vi "Create Object.vi"(8 "error in (no error)":errorcluster, 10 "Object Name":string, 11 "CS++Factory in":refnum<class "CS++Factory.lvclass">) -> (0 "error out":errorcluster, 1 "Attributes found?":bool, 2 "LabVIEW Object":refnum<class>, 3 "CS++Factory out":refnum<class "CS++Factory.lvclass">)   [LabVIEW 2013, in "CS++BaseClasses.lvlib" / "CS++Factory.lvclass"]
doc: "Create an object by name. Object name is a kind of reference to attribute initialization data."
uses:
  CS++Factory.lvclass
  Base/CS++Base.lvclass
  Actors/CS++BaseActor/CS++BaseActor.lvclass
  Actors/CS++BaseActor/CS++BaseActor.lvclass/CS++BaseActor.ctl
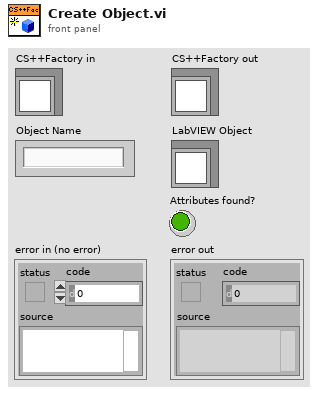
[diagram p1: front panel]
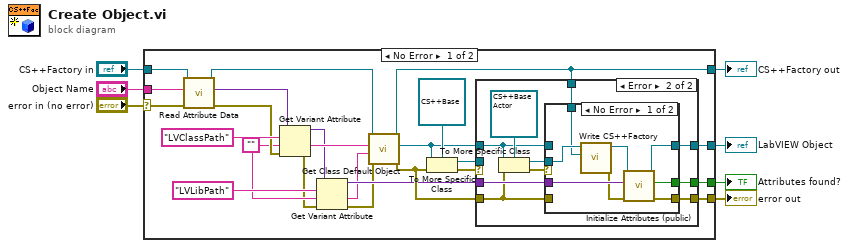
[diagram p0: block diagram]
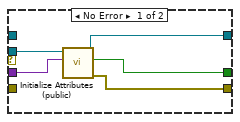
[diagram p2: hidden frame]
diagram:
  n1 = case shown="No Error" "error in (no error)" {
    selector: "error in (no error)" -> [w22 w58]
    tunnel: [w23 w58] -> w6
    tunnel: [w18 w57] -> w4
    tunnel: "CS++Factory in" -> [w31 w57]
    tunnel: [w24 _] -> w3
    tunnel: "Object Name" -> [w30 _]
    tunnel: [w21 _] -> w1
    frame No Error {
      w10 = ""
      n2 = call-dynamic "Read Attribute Data.vi"("error in (no error)"=w22, "Object Name"=w30, "CS++Factory in"=w31) -> ("error out"=w27:errorcluster, "Attribute Data"=w29:variant, "CS++Factory out"=w19:refnum<class "CS++Factory.lvclass">)  [unwired: 6 in]
      n3 = Get Variant Attribute(Variant=w29, name="LVClassPath", default value (empty Variant)=w10, error in=w27) -> (duplicate Variant=w13:variant, value=w16:string, error out=w9:errorcluster)  [unwired: 1 out]
      n4 = Get Variant Attribute(Variant=w13, name="LVLibPath", default value (empty Variant)=w10, error in=w9) -> (duplicate Variant=w12:variant, value=w11:string, error out=w8:errorcluster)  [unwired: 1 out]
      n5 = call-dynamic "Get Class Default Object.vi"("error in (no error)"=w8, "Library Path/Name"=w11, "Class Path/Name"=w16, "CS++Factory in"=w19) -> ("error out"=w17:errorcluster, "Class Default Object"=w15:refnum<class>, "CS++Factory out"=w18:refnum<class "CS++Factory.lvclass">)  [unwired: 5 in]
      n6 = To More Specific Class(target class=refnum<class "CS++Base.lvclass"> refnum ("CS++BaseClasses.lvlib:CS++Base.lvclass"), reference=w15, error in=w17) -> (specific class reference=w25:refnum<class "CS++Base.lvclass">, error out=w20:errorcluster)
      n7 = case shown="Error" w20 {
        tunnel: w25 -> [w36 _]
        tunnel: w12 -> [w35 w41]
        tunnel: [w34 w43] -> w24
        tunnel: [w33 w40] -> w23
        tunnel: [w32 w39] -> w21
        tunnel: w15 -> [_ w42]
        tunnel: w17 -> [_ w38]
        tunnel: w18 -> [_ w37]
        frame No Error {
          n8 = call "Initialize Attributes (public).vi"("Attribute Data"=w35, "CS++Base in"=w36) -> ("error out"=w33:errorcluster, "Found?"=w32:bool, "CS++Base out"=w34:refnum<class "CS++Base.lvclass">)  [unwired: 7 in]
        }
        frame Error {
          n9 = To More Specific Class(target class=refnum<class "CS++BaseActor.lvclass"> refnum ("CS++BaseActor.lvlib:CS++BaseActor.lvclass"), reference=w42, error in=w38) -> (specific class reference=w45:refnum<class "CS++BaseActor.lvclass">, error out=w44:errorcluster)
          n10 = case shown="No Error" w44 {
            tunnel: w45 -> [w54 _]
            tunnel: [w51 w56] -> w43
            tunnel: w42 -> [_ w56]
            tunnel: w41 -> [w50 _]
            tunnel: [w48 w55] -> w40
            tunnel: [w47 _] -> w39
            tunnel: w38 -> [_ w55]
            tunnel: w37 -> [w53 _]
            frame No Error {
              n11 = call "Write CS++Factory.vi"("CS++Factory"=w53, "CS++BaseActor in"=w54) -> ("error out"=w49:errorcluster, "CS++BaseActor out"=w52:refnum<class "CS++BaseActor.lvclass">)  [unwired: 8 in]
              n12 = call "Initialize Attributes (public).vi"("error in (no error)"=w49, "Attribute Data"=w50, "CS++BaseActor in"=w52) -> ("error out"=w48:errorcluster, "Found?"=w47:bool, "CS++BaseActor out"=w51:refnum<class "CS++BaseActor.lvclass">)  [unwired: 6 in]
            }
            frame Error {
            }
          }
        }
      }
    }
    frame Error {
    }
  }
  "error out" <- w6
  "CS++Factory out" <- w4
  "LabVIEW Object" <- w3
  "Attributes found?" <- w1
